vi "Panel Resized.vi"(6 "Sizing Refnums":T2, 8 "error in (no error)":errorcluster, 9 "Origin":cluster{"H":i16, "V":i16}, 10 "NewBnds":T1, 11 "Size Constraints":cluster{"min tab width":i32, "w/h":dbl}) -> (0 "error out":errorcluster)   [LabVIEW 2019]
uses:
  <vilib>/Utility/miscctls.llb/LVRectTypeDef.ctl
  <vilib>/Utility/miscctls.llb/LVRowAndColumnTypeDef.ctl
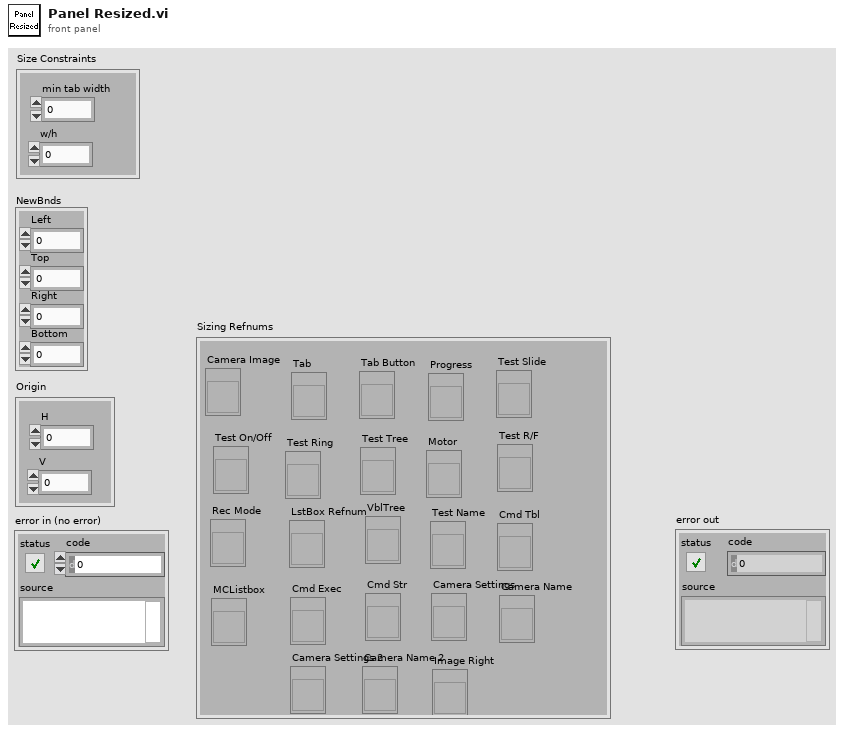
[diagram p1: front panel]
types:
  T1 = typedef "LVRectTypeDef.ctl" = cluster{"Left":i16, "Top":i16, "Right":i16, "Bottom":i16}
  T2 = cluster{"Camera Image":refnum<vi>, "Tab":refnum<vi>, "Tab Button":refnum<vi>, "Rec Mode":refnum<vi>, "Test Slide":refnum<vi>, "Test On/Off":refnum<vi>, "Test Ring":refnum<vi>, "Test R/F":refnum<vi>, "Test Name":refnum<vi>, "Motor":refnum<vi>, "Progress":refnum<vi>, "LstBox Refnum":refnum<vi>, "Test Tree":refnum<vi>, "VblTree":refnum<vi>, "Cmd Tbl":refnum<vi>, "MCListbox":refnum<vi>, "Cmd Exec":refnum<vi>, "Cmd Str":refnum<vi>, "Camera Settings":refnum<vi>, "Camera Name":refnum<vi>, "Camera Settings 2":refnum<vi>, "Camera Name 2":refnum<vi>, "Image Right":refnum<vi>}
  T3 = typedef "LVRowAndColumnTypeDef.ctl" = cluster{"Row":i32, "Column":i32}
  T4 = typedef "LVPositionTypeDef.ctl" = cluster{"Left":i32, "Top":i32}
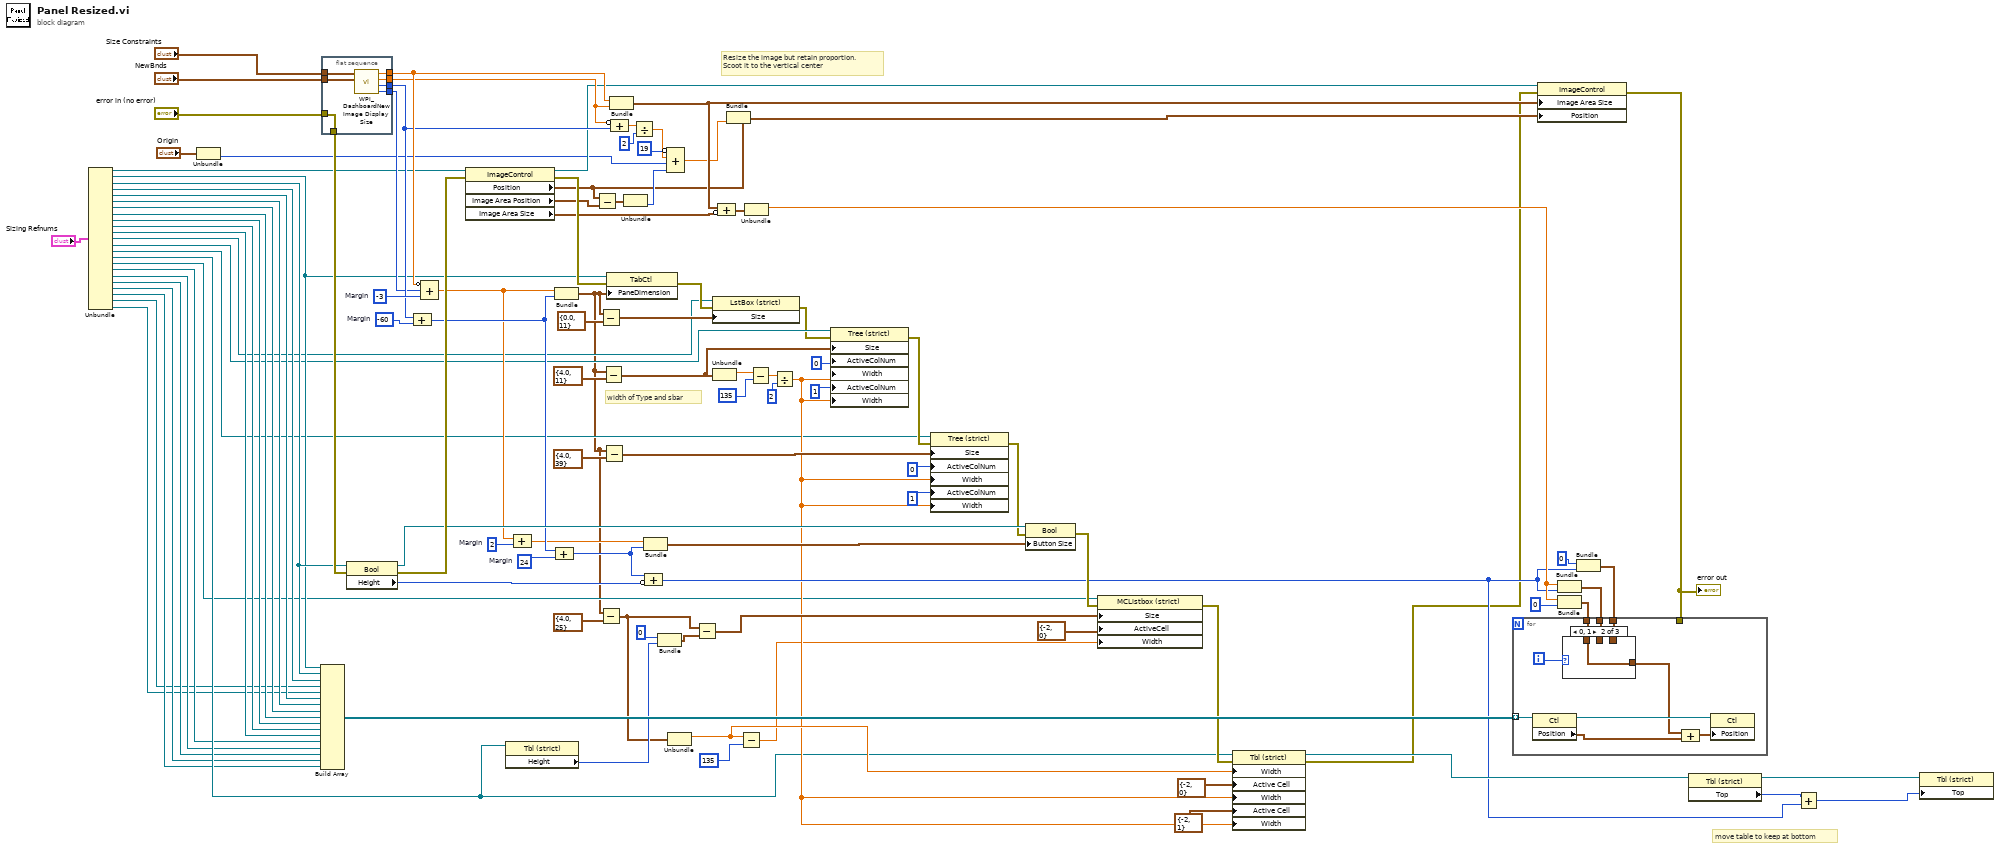
[diagram p0: block diagram]
diagram:
  w96 = 24  # Margin
  w94 = 2  # Margin
  w90 = -60  # Margin
  w100 = -3  # Margin
  # "move table to keep at bottom"
  # "width of Type and sbar"
  # "Resize the image but retain proportion.\nScoot it to the vertical center"
  n1 = Unbundle("Sizing Refnums") -> ("Camera Image"=w64:refnum<vi>, "Tab"=w65:refnum<vi>, "Tab Button"=w73:refnum<vi>, "Rec Mode"=w22:refnum<vi>, "Test Slide"=w21:refnum<vi>, "Test On/Off"=w20:refnum<vi>, "Test Ring"=w19:refnum<vi>, "Test R/F"=w18:refnum<vi>, "Test Name"=w17:refnum<vi>, "Motor"=w16:refnum<vi>, "Progress"=w15:refnum<vi>, "LstBox Refnum"=w14:refnum<vi>, "Test Tree"=w13:refnum<vi>, "VblTree"=w12:refnum<vi>, "Cmd Tbl"=w11:refnum<vi>, "MCListbox"=w10:refnum<vi>, "Cmd Exec"=w9:refnum<vi>, "Cmd Str"=w8:refnum<vi>, "Camera Settings"=w7:refnum<vi>, "Camera Name"=w6:refnum<vi>, "Camera Settings 2"=w5:refnum<vi>, "Camera Name 2"=w4:refnum<vi>, "Image Right"=w3:refnum<vi>)
  n2 = Unbundle("Origin") -> ("V"=w70:i16)  [unwired: 1 out]
  n3 = Build Array(w65, w73, w22, w4, w3, w21, w20, w19, w18, w17, w16, w15, w9, w8, w7, w6, w5) -> (w109:refnum<vi>[])
  n4 = flat-sequence {
    tunnel: "NewBnds" -> [w116]
    tunnel: "Size Constraints" -> [w115]
    tunnel: [w114] -> w89
    tunnel: [w113] -> w97
    tunnel: [w112] -> w98
    tunnel: [w111] -> w99
    tunnel: [w110] -> w108
    tunnel: "error in (no error)" -> [w110]
    frame #0 {
      n5 = call <vilib>:"WPI_DashboardNew Image Display Size.vi"("NewBnds"=w116, "Size Constraints"=w115) -> ("Window Width"=w114:i16, "Window Height"=w112:i16, "Height"=w113:dbl, "Width"=w111:dbl)  [unwired: 6 in]
    }
  }
  n6 = property class="Bool"(reference=w73, error in=w108) -> (reference out=w103:refnum<vi>, error out=w107:errorcluster, "Height"=w102:u32)
  n7 = Compound Arithmetic op=unknown(w98, w90) -> (w95:i32)
  n8 = Compound Arithmetic op=ADD(invert w99, w89, w100) -> (w93:dbl)
  n9 = property class="ImageControl"(reference=w64, error in=w107) -> (reference out=w82:refnum<vi>, error out=w106:errorcluster, "Position"=w81:T4, "Image Area Position"=w76:cluster{"Left":i32, "Top":i32}, "Image Area Size"=w87:cluster{"Width":u32, "Height":u32})
  n10 = property class="Tbl (strict)"(reference=w11) -> ("Height"=w40:u32)  [unwired: 1 in, 2 out]
  n11 = Compound Arithmetic op=ADD(w93, w94) -> (w92:dbl)
  n12 = Bundle(w93, w95) -> (w2:cluster{dbl, i32})  [unwired: 1 in]
  n13 = Compound Arithmetic op=ADD(w95, w96) -> (w101:i32)
  n14 = Subtract(x=w81, y=w76) -> (x-y=w83:T4)
  n15 = Subtract(x=w2, y=cluster{dbl, i32} {0.0, 11}) -> (x-y=w62:cluster{dbl, i32})
  n16 = Subtract(x=w2, y=cluster{dbl, i32} {4.0, 25}) -> (x-y=w37:cluster{dbl, i32})
  n17 = Subtract(x=w2, y=cluster{dbl, i32} {4.0, 11}) -> (x-y=w53:cluster{dbl, i32})
  n18 = Subtract(x=w2, y=cluster{dbl, i32} {4.0, 39}) -> (x-y=w58:cluster{dbl, i32})
  n19 = property class="TabCtl"(reference=w65, error in=w106, "PaneDimension"=w2) -> (error out=w63:errorcluster)  [unwired: 1 out]
  n20 = Bundle("Width"=w99, "Height"=w97) -> (w85:cluster{"Width":dbl, "Height":dbl})  [unwired: 1 in]
  n21 = Compound Arithmetic op=ADD(invert w97, w98) -> (w77:dbl)
  n22 = Unbundle(w83) -> ("Top"=w84:i32)  [unwired: 1 out]
  n23 = Divide(x=w77, y=2) -> (x/y=w79:dbl)
  n24 = Bundle(w92, w101) -> (w91:cluster{dbl, i32})  [unwired: 1 in]
  n25 = Compound Arithmetic op=ADD(w101, invert w102) -> (w32:u32)
  n26 = Bundle(0, "Height"=w40) -> (w38:cluster{i32, "Height":u32})  [unwired: 1 in]
  n27 = Compound Arithmetic op=ADD(invert 19, w79, w70, w84) -> (w80:dbl)
  n28 = Unbundle(w37) -> (w27:dbl)  [unwired: 1 out]
  n29 = Subtract(x=w37, y=w38) -> (x-y=w36:cluster{dbl, u32})
  n30 = property class="LstBox (strict)"(reference=w14, error in=w63, "Size"=w62) -> (error out=w1:errorcluster)  [unwired: 1 out]
  n31 = Unbundle(w53) -> (w52:dbl)  [unwired: 1 out]
  n32 = Compound Arithmetic op=ADD(w85, invert w87) -> (w88:cluster{"Width":dbl, "Height":dbl})
  n33 = Bundle(cluster=w81, "Top"=w80) -> (w86:T4)  [unwired: 1 in]
  n34 = Subtract(x=w27, y=135) -> (x-y=w24:dbl)
  n35 = Unbundle(w88) -> ("Width"=w104:dbl)  [unwired: 1 out]
  n36 = Subtract(x=w52, y=135 ("Active Cell:Active Column Number")) -> (x-y=w48:dbl)
  n37 = Divide(x=w48, y=2 ("Active Cell:Active Column Number")) -> (x/y=w25:dbl)
  n38 = property class="Tree (strict)"(reference=w13, error in=w1, "Size"=w53, "ActiveColNum"=0 ("Active Cell:Active Column Number"), "Width"=w25, "ActiveColNum"=1 ("Active Cell:Active Column Number"), "Width"=w25) -> (error out=w57:errorcluster)  [unwired: 1 out]
  n39 = property class="Tree (strict)"(reference=w12, error in=w57, "Size"=w58, "ActiveColNum"=0 ("Active Cell:Active Column Number"), "Width"=w25, "ActiveColNum"=1 ("Active Cell:Active Column Number"), "Width"=w25) -> (error out=w56:errorcluster)  [unwired: 1 out]
  n40 = property class="Bool"(reference=w103, error in=w56, "Button Size"=w91) -> (error out=w44:errorcluster)  [unwired: 1 out]
  n41 = property class="MCListbox (strict)"(reference=w10, error in=w44, "Size"=w36, "ActiveCell"=T3 {"Row"=-2, "Column"=0} ("Active Cell:Active Cell"), "Width"=w24) -> (error out=w41:errorcluster)  [unwired: 1 out]
  n42 = property class="Tbl (strict)"(reference=w11, error in=w41, "Width"=w27, "Active Cell"=T3 {"Row"=-2, "Column"=0} ("Active Cell:Active Cell"), "Width"=w25, "Active Cell"=T3 {"Row"=-2, "Column"=1} ("Active Cell:Active Cell"), "Width"=w25) -> (reference out=w35:refnum<vi>, error out=w30:errorcluster)
  n43 = property class="ImageControl"(reference=w82, error in=w30, "Image Area Size"=w85, "Position"=w86) -> (error out=w69:errorcluster)  [unwired: 1 out]
  "error out" <- w69
  n44 = Bundle("Width"=w104, w32) -> (w75:cluster{"Width":dbl, u32})  [unwired: 1 in]
  n45 = Bundle("Width"=w104, 0) -> (w74:cluster{"Width":dbl, i32})  [unwired: 1 in]
  n46 = Bundle(0, w32) -> (w45:cluster{i32, u32})  [unwired: 1 in]
  n47 = for {
    tunnel: w109 -> [w125] mode=indexing
    tunnel: w75 -> [w119]
    tunnel: w74 -> [w120]
    tunnel: w69 -> [_]
    tunnel: w45 -> [w118]
    i -> [w121]
    n48 = property class="Ctl"(reference=w125) -> (reference out=w124:refnum<vi>, "Position"=w123:T4)  [unwired: 1 in, 1 out]
    n49 = case shown="0, 1" w121 {
      tunnel: w120 -> [_ w127 _]
      tunnel: w119 -> [_ _ w128]
      tunnel: w118 -> [w126 _ _]
      tunnel: [w126 w127 w128] -> w117
      frame Default {
      }
      frame 0, 1 {
      }
      frame 2..4 {
      }
    }
    n50 = Compound Arithmetic op=ADD(w117, w123) -> (w122:cluster{dbl, u32})
    n51 = property class="Ctl"(reference=w124, "Position"=w122) -> ()  [unwired: 1 in, 2 out]
  }
  n52 = property class="Tbl (strict)"(reference=w35) -> (reference out=w34:refnum<vi>, "Top"=w33:i32)  [unwired: 1 in, 1 out]
  n53 = Add(x=w33, y=w32) -> (x+y=w31:u32)
  n54 = property class="Tbl (strict)"(reference=w34, "Top"=w31) -> ()  [unwired: 1 in, 2 out]
